vi "GOMDBTS2048 calib Set Calibration Factors Spectral.vi"(8 "error in (no error)":errorcluster, 10 "values":dbl[](array[numeric]), 11 "handle":i32) -> (0 "error out":errorcluster, 3 "function return":i32)   [LabVIEW 2015, in "GOMDBTS2048.lvlib"]
doc: "GOBTS2048DLL int __stdcall GOMDBTS2048_calibAzSetWeightingFunctionActual(int handle, double* values); GOBTS2048DLL int __stdcall GOMDBTS2048_calibAzGetWeightingFunctionActual(int handle, double* values); GOBTS2048DLL int __stdcall GOMDBTS2048_calibSetCalibrationFactorsSpectral(int handle, double* values);"
uses:
  GOMDBTS2048.lvlib
  runtime/GOMDBTS2048.dll
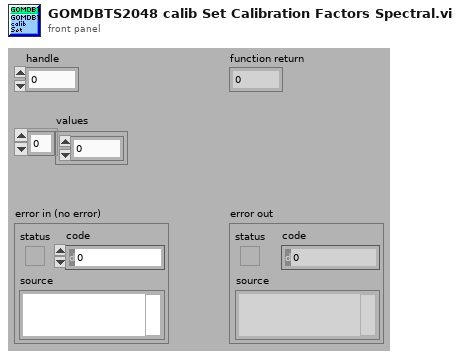
[diagram p1: front panel]
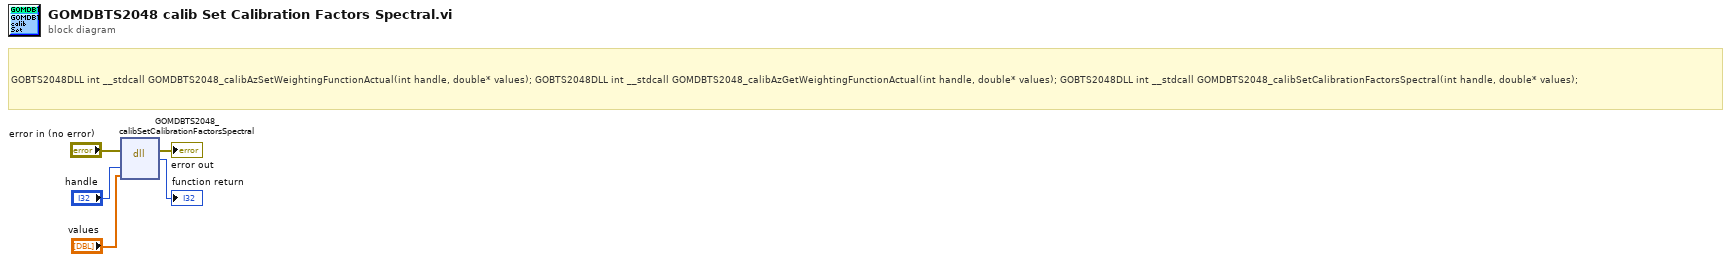
[diagram p0: block diagram]
diagram:
  # "GOBTS2048DLL int __stdcall GOMDBTS2048_calibAzSetWeightingFunctionActual(int handle, double* values); GOBTS2048DLL int __stdcall GOMDBTS2048_calibAzGetWeightingFunctionActual(int handle, double* values); GOBTS2048DLL int __stdcall GOMDBTS2048_calibSetCalibrationFactorsSpectral(int handle, double* values);"
  n1 = dll-call lib="C:/Users/rkoch/Documents/GO_Library/runtime/GOMDBTS2048.*" fn="GOMDBTS2048_calibSetCalibrationFactorsSpectral"(error in="error in (no error)", "handle"="handle", "values"="values") -> (error out=→"error out":errorcluster, →"function return":i32)  [unwired: 4 in, 1 out]
